vi "Query Series.vi"(0 "InfluxDB in":refnum<class "Client.lvclass">, 5 "Database name":string, 7 "Measurement query":string, 9 "Precision":T1=enum."Nanoseconds", 11 "error in (no error)":errorcluster, 12 "Chunk size":i32) -> (4 "InfluxDB out":refnum<class "Client.lvclass">, 6 "Results Out":refnum<class "Results.lvclass">, 15 "error out":errorcluster)   [LabVIEW 2018, in "InfluxDB Client.lvlib" / "Client.lvclass"]
doc: "Creates a database."
uses:
  Client.lvclass
  Results/Results.lvclass
  Controls/Precision.ctl
  <vilib>/LVH/i3 JSON/i3-json.lvlib
  InfluxDB Client.lvlib
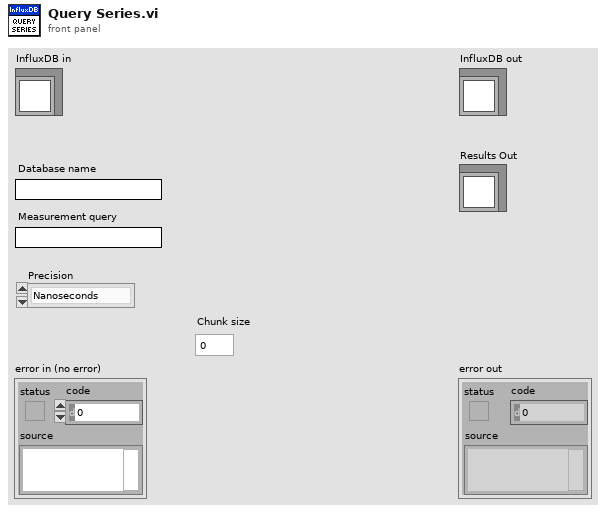
[diagram p1: front panel]
types:
  T1 = typedef "InfluxDB Client.lvlib/Precision.ctl" = enum16{"Seconds", "Milliseconds", "Nanoseconds"}
  T2 = typedef "Dictionary Object RefNum__ogtk.ctl" = refnum<k1>
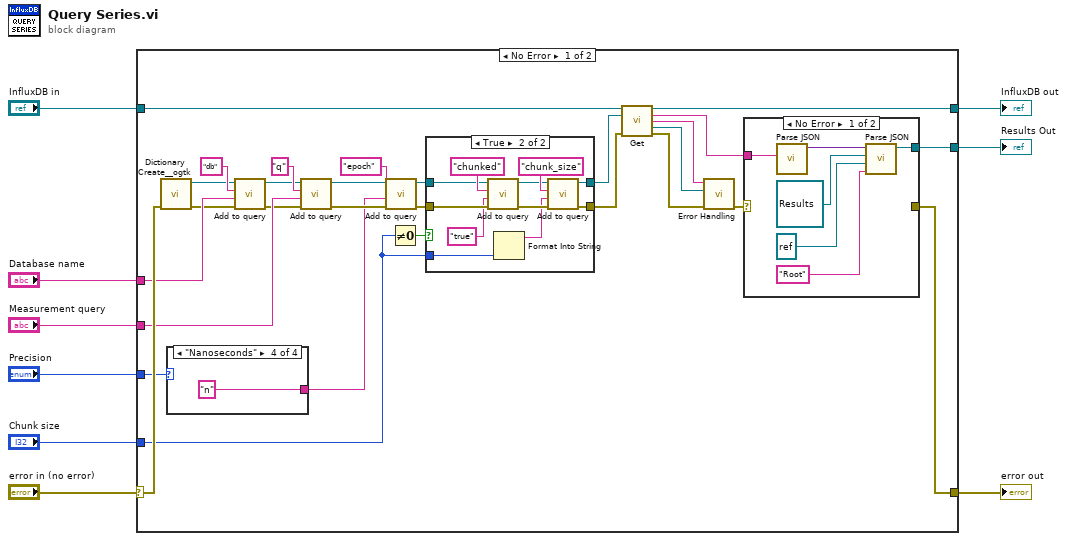
[diagram p0: block diagram]
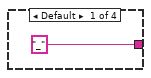
[diagram p4: hidden frame]
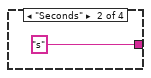
[diagram p5: hidden frame]
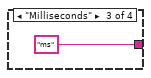
[diagram p6: hidden frame]
diagram:
  n1 = case shown="No Error" "error in (no error)" {
    selector: "error in (no error)" -> [w35 w64]
    tunnel: [w12 w64] -> w8
    tunnel: [w37 w63] -> w6
    tunnel: "InfluxDB in" -> [w38 w63]
    tunnel: [w10 _] -> w5
    tunnel: "Database name" -> [w33 _]
    tunnel: "Measurement query" -> [w32 _]
    tunnel: "Precision" -> [w30 _]
    tunnel: "Chunk size" -> [w21 _]
    frame No Error {
      n2 = call <userlib>:"Dictionary Create__ogtk.vi"("error in (no error)"=w35) -> ("error out"=w27:errorcluster, "dictionary out"=w28:T2)  [unwired: 9 in]
      n3 = case shown="\"Nanoseconds\"" w30 {
        tunnel: ["_" "s" "ms" "n"] -> w23
        frame Default {
        }
        frame "Seconds" {
        }
        frame "Milliseconds" {
        }
        frame "Nanoseconds" {
        }
      }
      n4 = call "Add to query.vi"("error in (no error)"=w27, "Value"=w33, "Parameter"="db" ("String"), "Query in"=w28) -> ("error out"=w26:errorcluster, "Query out"=w29:T2)  [unwired: 6 in]
      n5 = call "Add to query.vi"("error in (no error)"=w26, "Value"=w32, "Parameter"="q" ("String"), "Query in"=w29) -> ("error out"=w25:errorcluster, "Query out"=w24:T2)  [unwired: 6 in]
      n6 = call "Add to query.vi"("error in (no error)"=w25, "Value"=w23, "Parameter"="epoch" ("String"), "Query in"=w24) -> ("error out"=w17:errorcluster, "Query out"=w19:T2)  [unwired: 6 in]
      n7 = Not Equal To 0?(x=w21) -> (x != 0?=w22:bool)
      n8 = case shown="True" w22 {
        tunnel: w21 -> [_ w49]
        tunnel: [w47 w53] -> w20
        tunnel: w19 -> [w47 w51]
        tunnel: [w46 w54] -> w18
        tunnel: w17 -> [w46 w56]
        frame False {
        }
        frame True {
          n9 = call "Add to query.vi"("error in (no error)"=w56, "Value"="true" ("String"), "Parameter"="chunked" ("String"), "Query in"=w51) -> ("error out"=w55:errorcluster, "Query out"=w52:T2)  [unwired: 6 in]
          n10 = Format Into String(w49) -> (resulting string=w48:string)  [unwired: 3 in, 1 out]
          n11 = call "Add to query.vi"("error in (no error)"=w55, "Value"=w48, "Parameter"="chunk_size" ("String"), "Query in"=w52) -> ("error out"=w54:errorcluster, "Query out"=w53:T2)  [unwired: 6 in]
        }
      }
      n12 = call "Get.vi"("InfluxDB Client in"=w38, "Query"=w20, "error in (no error)"=w18) -> ("InfluxDB Client out"=w37:refnum<class "Client.lvclass">, "body"=w11:string, "Status code"=w16:string, "Headers"=w15:T2, "error out"=w13:errorcluster)  [unwired: 8 in]
      n13 = call "Error Handling.vi"("error in (no error)"=w13, "HTTP headers"=w15, "HTTP status code"=w16) -> ("error out"=w14:errorcluster)  [unwired: 8 in]
      n14 = case shown="No Error" w14 {
        selector: w14 -> [_ w45]
        tunnel: [_ w45] -> w12
        tunnel: w11 -> [w40 _]
        tunnel: [w39 _] -> w10
        frame No Error {
          n15 = call <vilib>:"Parse JSON.vi"("JSON String"=w40) -> ("JSON Tree"=w44:variant)  [unwired: 7 in, 3 out]
          n16 = call <vilib>:"Parse JSON.vi"("Path"="Root", "Log File Ref"=refnum<file> refnum, "Results In"=refnum<class "Results.lvclass"> refnum, "JSON Tree"=w44) -> ("Results Out"=w39:refnum<class "Results.lvclass">)  [unwired: 7 in]
        }
        frame Error {
        }
      }
    }
    frame Error {
    }
  }
  "error out" <- w8
  "InfluxDB out" <- w6
  "Results Out" <- w5
